vi "GetLanguageMode.vi"(8 "error in":errorcluster, 11 "VISA resource name":refnum<visa-resource-name>) -> (0 "error out":errorcluster, 1 "Language Mode Integer":i32, 2 "Language Mode string":string, 3 "VISA resource name out":refnum<visa-resource-name>)   [LabVIEW 2023, in "Thermotron 8800.lvlib"]
doc: "LANG\nCommand name: Send language mode\nCommand type: System status\nDescription: This command queries the 8800 for the current language mode.\nSyntax: LANG?\nThe 8800 will respond with 0 (English) or 1 (French).\nData type: Integer\nQuery example: LANG?\n8800 response: 1 (The 8800 is in French language mode.)"
uses:
  Thermotron 8800.lvlib
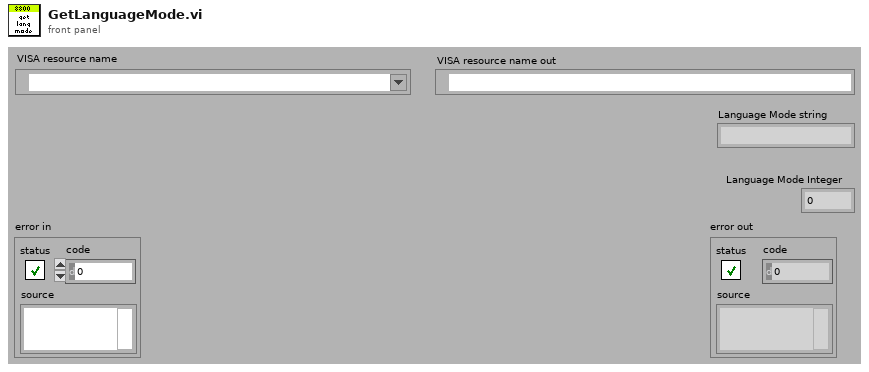
[diagram p1: front panel]
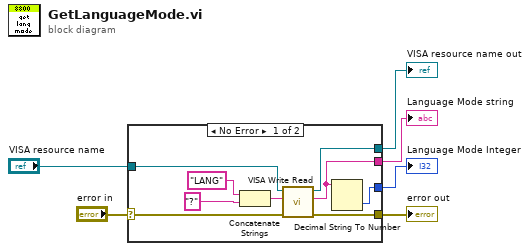
[diagram p0: block diagram]
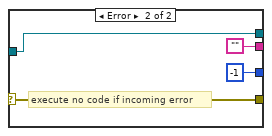
[diagram p2: hidden frame]
diagram:
  n1 = case shown="No Error" "error in" {
    selector: "error in" -> [w14 w19]
    tunnel: [w12 w19] -> w3
    tunnel: [w13 w18] -> w4
    tunnel: "VISA resource name" -> [w10 w18]
    tunnel: [w8 ""] -> w2
    tunnel: [w7 -1] -> w1
    frame No Error {
      n2 = Concatenate Strings("LANG" ("8800 Command"), "?" ("8800 Command")) -> (w15:string)
      n3 = call "VISA Write Read.vi"("error in (no error)"=w14, "8800 Command"=w15, "VISA Refnum in"=w10) -> ("error out"=w12:errorcluster, "read buffer"=w8:string, "VISA Refnum out"=w13:refnum<visa-resource-name>)  [unwired: 6 in]
      n4 = Decimal String To Number(string=w8) -> (number=w7:i32)  [unwired: 2 in, 1 out]
    }
    frame Error {
      # "execute no code if incoming error"
    }
  }
  "VISA resource name out" <- w4
  "error out" <- w3
  "Language Mode string" <- w2
  "Language Mode Integer" <- w1
